vi "NI6363_CreateTasks.vi"(0 "tasks in":refnum<k21>[](array[refnum]), 1 "Camera Trigger":string="Dev1/ctr0", 2 "Exposure (s)":dbl=0.1 min=1.0 max=5000.0, 5 "Dye Settings":T1={"Dye Name"="", "Pulse Sequence"=[], "Emission Filter"=0, "Exposure (s)"=0.01, "Yellow Select"=FALSE, "# Pulses"=0} {"Exposure (s)" min=1.0 max=5000.0}, 7 "Sample Mode":T2(ring), 9 "Number of Samples":i32=100, 11 "error in":errorcluster) -> (4 "tasks out":refnum<k21>[](array[refnum]), 10 "Seq Length (s)":dbl, 15 "error out":errorcluster)   [LabVIEW 2010]
uses:
  <vilib>/DAQmx/write.llb/DAQmx Write (Digital 2D U32 NChan NSamp).vi
  <vilib>/DAQmx/write.llb/DAQmx Write (Analog 2D DBL NChan NSamp).vi
  <vilib>/daqmx/miscellaneous.llb/DAQmx Fill In Error Info.vi
  <vilib>/DAQmx/configure/trigger.llb/DAQmx Start Trigger (None).vi
  <vilib>/DAQmx/configure/timing.llb/DAQmx Timing (Implicit).vi
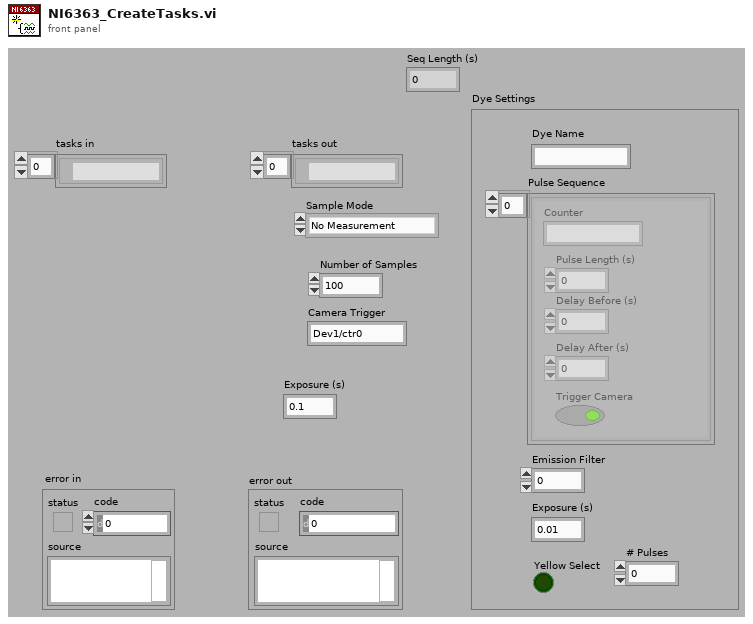
[diagram p1: front panel]
types:
  T1 = cluster{"Dye Name":string, "Pulse Sequence":cluster{"Counter":string, "Pulse Length (s)":dbl, "Delay Before (s)":dbl, "Delay After (s)":dbl, "Trigger Camera":bool}[], "Emission Filter":i16, "Exposure (s)":dbl, "Yellow Select":bool, "# Pulses":i32}
  T2 = enum16{"No Measurement", "Single Sample", "Continuous Samples", "N Samples"}
  T3 = cluster{"Counter":string, "Pulse Length (s)":dbl, "Delay Before (s)":dbl, "Delay After (s)":dbl, "Trigger Camera":bool}[]
  T4 = cluster{"Counter":string, "Pulse Length (s)":dbl, "Delay Before (s)":dbl, "Delay After (s)":dbl, "Trigger Camera":bool}
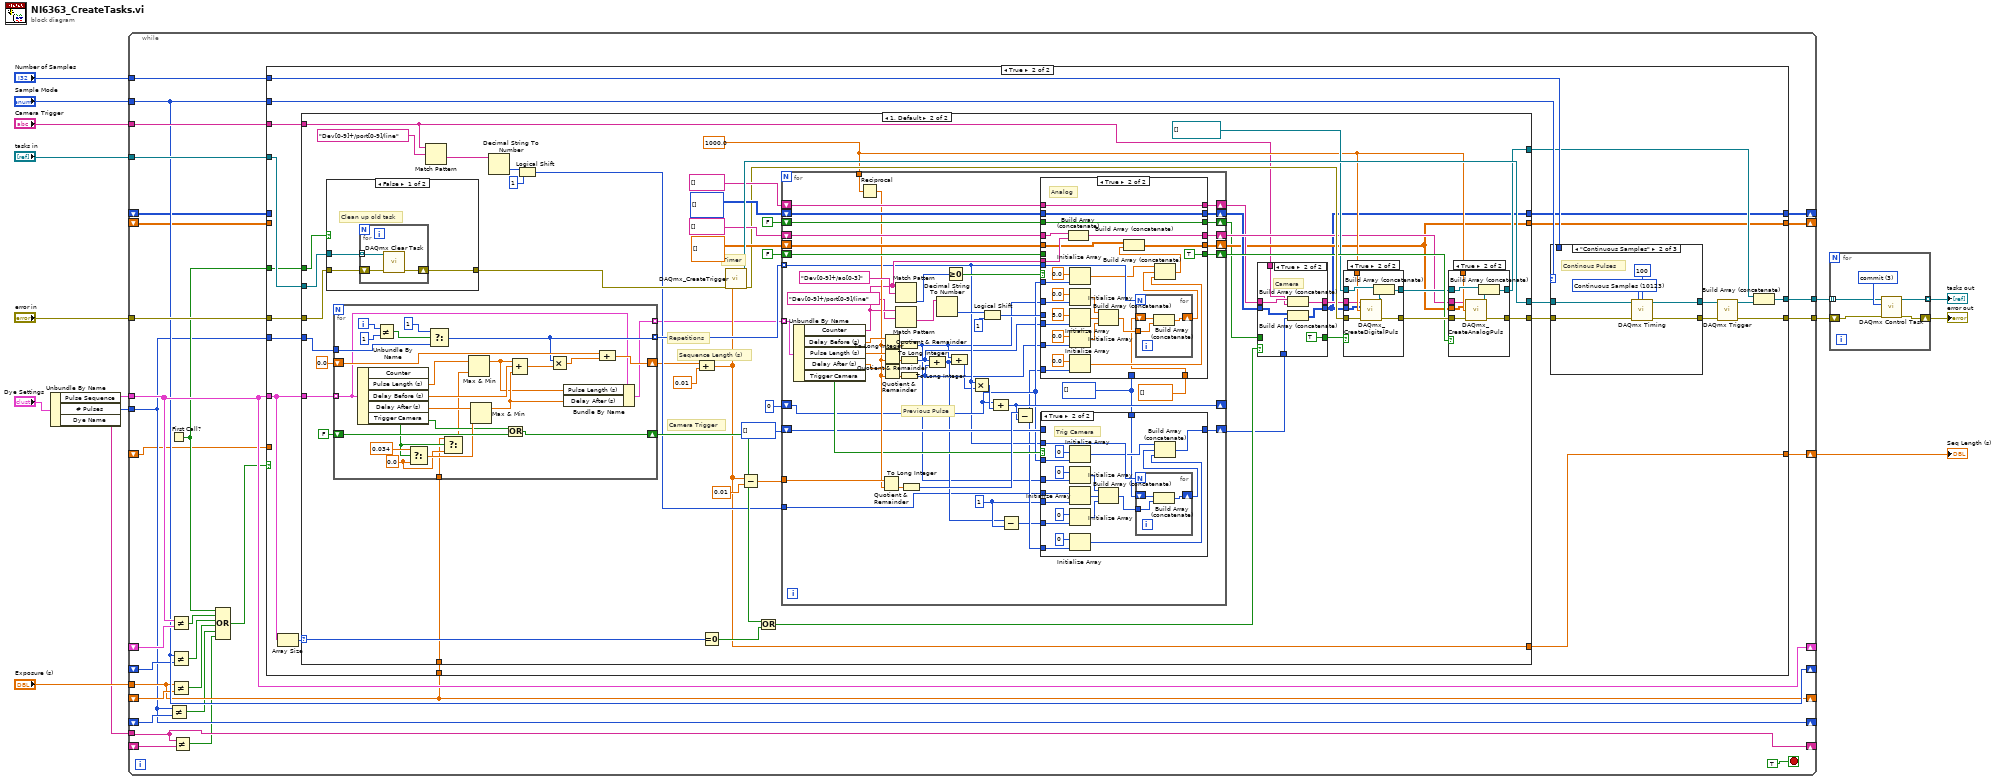
[diagram p0: block diagram]
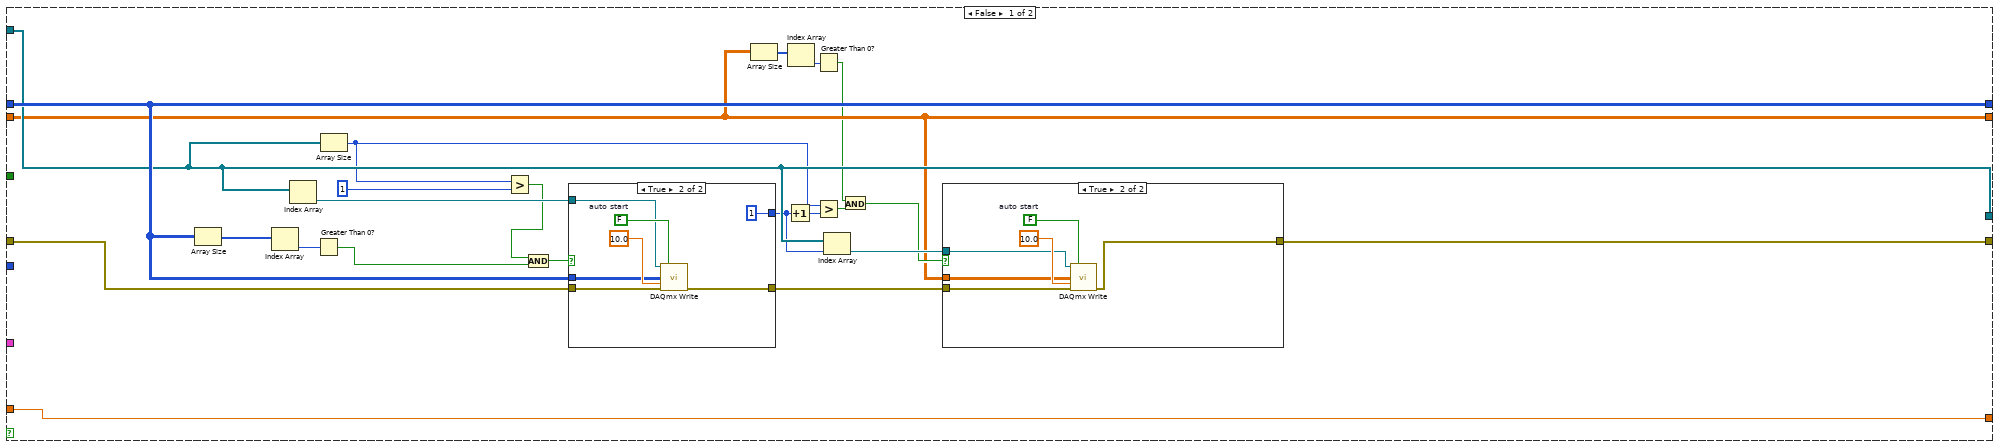
[diagram p2: hidden frame]
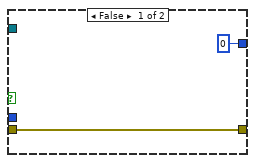
[diagram p4: hidden frame]
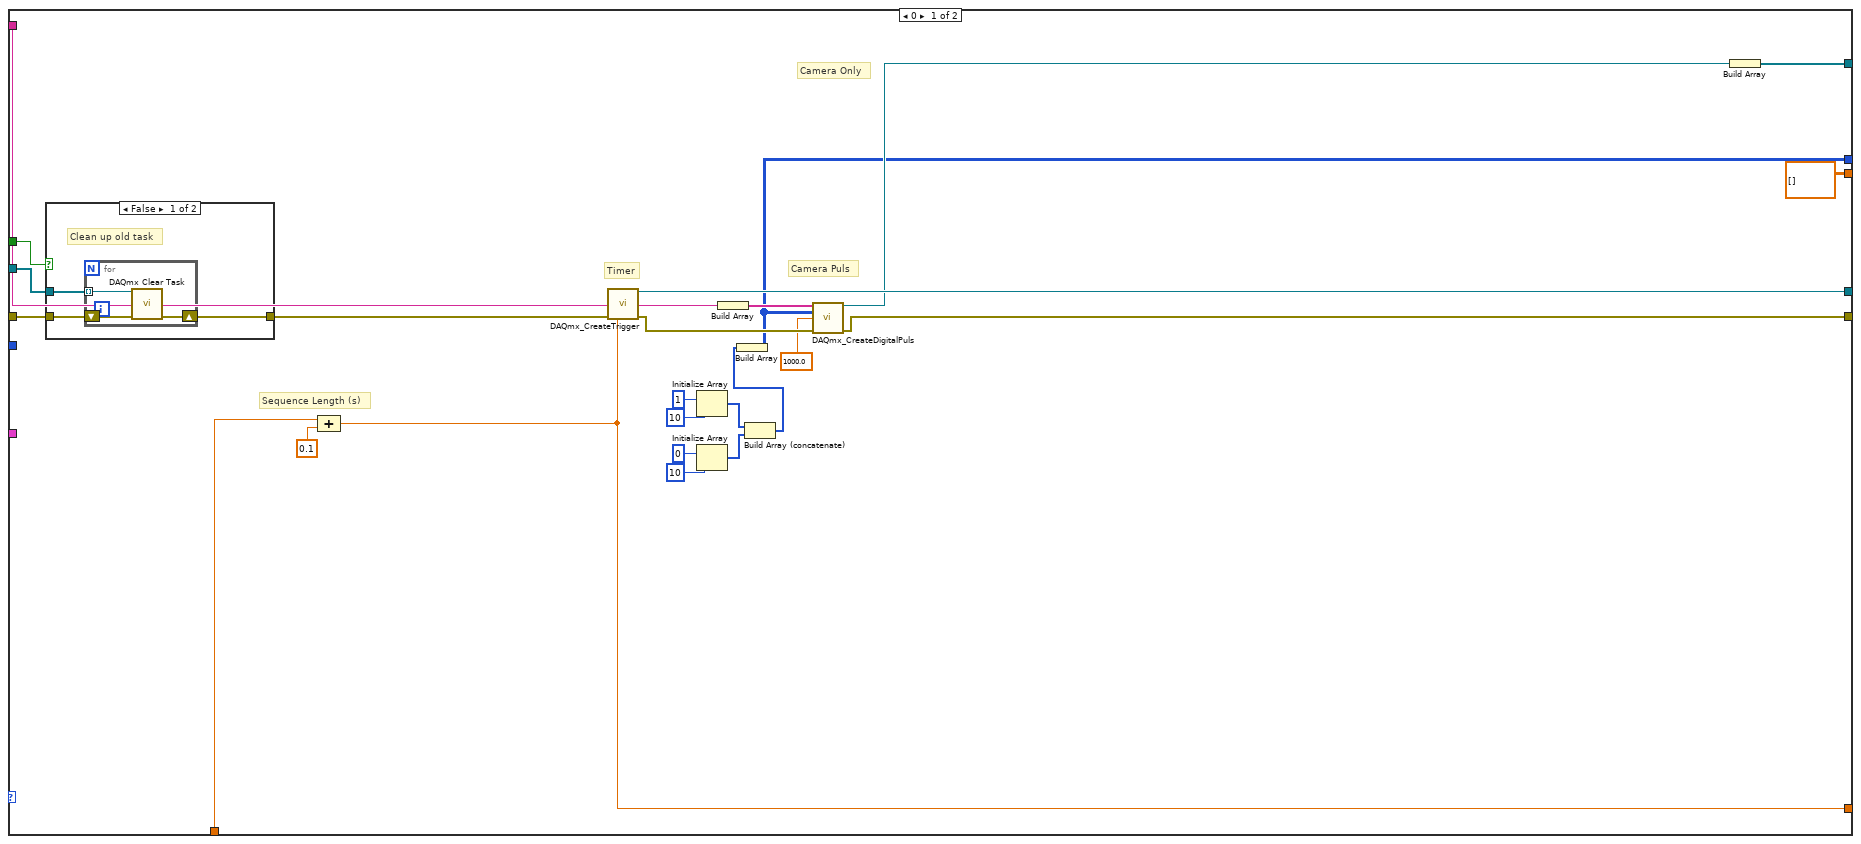
[diagram p5: hidden frame]
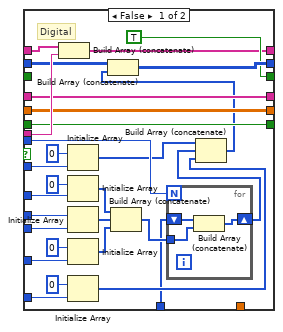
[diagram p12: hidden frame]
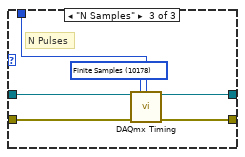
[diagram p14: hidden frame]
diagram:
  n1 = Unbundle By Name("Dye Settings") -> ("Pulse Sequence"=w9:T3, "# Pulses"=w8:i32, "Dye Name"=w2:string)
  n2 = while {
    tunnel: w9 -> [w38]
    tunnel: "Number of Samples" -> [w43]
    tunnel: "Camera Trigger" -> [w42]
    tunnel: "Sample Mode" -> [w33]
    tunnel: "error in" -> [w40]
    tunnel: [w44] -> w5
    tunnel: [w45] -> w6
    shift-right: [w38] -> _
    shift-left: _ -> [w39]
    tunnel: "tasks in" -> [w37]
    shift-right: [w33] -> _
    shift-left: _ -> [w32]
    tunnel: "Exposure (s)" -> [w29]
    shift-right: [w29] -> _
    shift-left: _ -> [w30]
    tunnel: w8 -> [w26]
    shift-right: [w26] -> _
    shift-left: _ -> [w28]
    shift-right: [w24] -> _
    shift-left: _ -> [w22]
    shift-right: [w23] -> _
    shift-left: _ -> [w21]
    tunnel: w2 -> [w19]
    shift-right: [w19] -> _
    shift-left: _ -> [w20]
    shift-right: [w17] -> w1
    shift-left: _ -> [w16]
    stop <- TRUE stop-if-true
    n3 = First Call?() -> (First Call?: T/F=w35:bool)
    n4 = Not Equal?(x=w26, y=w28) -> (x != y?=w27:bool)
    n5 = Not Equal?(x=w38, y=w39) -> (x != y?=w36:bool)
    n6 = Not Equal?(x=w33, y=w32) -> (x != y?=w34:bool)
    n7 = Not Equal?(x=w29, y=w30) -> (x != y?=w31:bool)
    n8 = Not Equal?(x=w19, y=w20) -> (x != y?=w18:bool)
    n9 = Compound Arithmetic op=OR(w35, w36, w34, w31, w27, w18) -> (w25:bool)
    n10 = case shown="True" w25 {
      tunnel: [w60 w91] -> w45
      tunnel: [w47 w103] -> w44
      tunnel: w43 -> [_ w102]
      tunnel: w42 -> [_ w100]
      tunnel: w33 -> [_ w99]
      tunnel: w40 -> [w68 w98]
      tunnel: w38 -> [_ w95]
      tunnel: w37 -> [w60 w97]
      tunnel: w35 -> [_ w96]
      tunnel: w29 -> [_ w94]
      tunnel: w26 -> [_ w92]
      tunnel: [w67 w87] -> w24
      tunnel: [w49 w86] -> w23
      tunnel: w22 -> [w67 _]
      tunnel: w21 -> [w49 _]
      tunnel: [w46 w85] -> w17
      tunnel: w16 -> [w46 _]
      frame False {
        n11 = Array Size(array=w67) -> (size(s)=w66:i32[])
        n12 = Index Array(array=w66) -> (element=w65:i32)  [unwired: 1 in]
        n13 = Index Array(array=w60) -> (element=w61:refnum<k21>)  [unwired: 1 in]
        n14 = Greater Than 0?(x=w65) -> (x > 0?=w64:bool)
        n15 = Array Size(array=w60) -> (size(s)=w55:i32)
        n16 = Greater?(x=w55, y=1) -> (0:w56:bool)
        n17 = And(x=w56, y=w64) -> (x .and. y?=w63:bool)
        n18 = case shown="True" w63 {
          tunnel: w68 -> [w77 w82]
          tunnel: w67 -> [_ w81]
          tunnel: [w77 w80] -> w62
          tunnel: [0 ("y") 1 ("y")] -> w53
          tunnel: w61 -> [_ w78]
          frame False {
          }
          frame True {
            w84 = FALSE  # auto start
            n19 = call-poly <vilib>:"DAQmx Write.vi"("task/channels in"=w78, "auto start"=w84, "data"=w81, "timeout"=10.0 ("timeout (s)"), "error in"=w82) -> ("error out"=w80:errorcluster)  [unwired: 8 in, 2 out]
          }
        }
        n20 = Array Size(array=w49) -> (size(s)=w51:i32[])
        n21 = Increment(x=w53) -> (x+1=w52:i32)
        n22 = Index Array(array=w51) -> (element=w50:i32)  [unwired: 1 in]
        n23 = Greater Than 0?(x=w50) -> (x > 0?=w48:bool)
        n24 = Greater?(x=w55, y=w52) -> (0:w58:bool)
        n25 = Index Array(array=w60, index=w53) -> (element=w59:refnum<k21>)
        n26 = And(x=w48, y=w58) -> (x .and. y?=w57:bool)
        n27 = case shown="True" w57 {
          tunnel: w62 -> [w69 w73]
          tunnel: w49 -> [_ w72]
          tunnel: w59 -> [_ w71]
          tunnel: [w69 w70] -> w47
          frame False {
          }
          frame True {
            w75 = FALSE  # auto start
            n28 = call-poly <vilib>:"DAQmx Write.vi"("task/channels in"=w71, "auto start"=w75, "data"=w72, "timeout"=10.0 ("timeout (s)"), "error in"=w73) -> ("error out"=w70:errorcluster)  [unwired: 8 in, 2 out]
          }
        }
      }
      frame True {
        n29 = Array Size(array=w95) -> (size(s)=w93:i32)
        n30 = case shown="1, Default" w93 {
          selector: w93 -> [_ w180]
          tunnel: [w110 w176] -> w101
          tunnel: w100 -> [w122 w145]
          tunnel: w98 -> [w129 w185]
          tunnel: w97 -> [w128 w184]
          tunnel: w96 -> [w127 w183]
          tunnel: w95 -> [_ w138]
          tunnel: w94 -> [w125 w139]
          tunnel: w92 -> [_ w152]
          tunnel: [w113 w178] -> w90
          tunnel: [w111 w165] -> w89
          tunnel: [w108 w155] -> w87
          tunnel: [dbl[][] [] w158] -> w86
          tunnel: [w106 w140] -> w85
          frame 0 {
            # "Timer"
            # "Camera Only"
            # "Camera Puls"
            # "Sequence Length (s)"
            n31 = case shown="False" w127 {
              tunnel: w129 -> [w131 w136]
              tunnel: [w132 w136] -> w124
              tunnel: w128 -> [w130 _]
              frame False {
                # "Clean up old task"
                n32 = for {
                  tunnel: w130 -> [w133] mode=indexing
                  shift-right: [w135] -> w132
                  shift-left: w131 -> [w134]
                  n33 = call <vilib>:"DAQmx Clear Task.vi"("task in"=w133, "error in"=w134) -> ("error out"=w135:errorcluster)  [unwired: 13 in]
                }
              }
              frame True {
              }
            }
            n34 = Compound Arithmetic op=ADD(w125, 0.1 ("Delay After (s) 2")) -> (w106:dbl)
            n35 = call "DAQmx_CreateTrigger.vi"("error in"=w124, "Sequence Length (s)"=w106) -> ("task out"=w113:refnum<k21>, "error out"=w123:errorcluster)  [unwired: 12 in]
            n36 = Initialize Array(u32 1 ("element"), 10 ("dimension size")) -> (w116:u32[])
            n37 = Initialize Array(u32 0 ("element"), 10 ("dimension size")) -> (w115:u32[])
            n38 = Build Array(w122) -> (w121:string[])
            n39 = Build Array (concatenate)(w116, w115) -> (w109:u32[])
            n40 = Build Array(w109) -> (w108:u32[][])
            n41 = call "DAQmx_CreateDigitalPuls.vi"("lines"=w121, "data"=w108, "rate"=1000.0, "error in"=w123) -> ("task out"=w112:refnum<k21>, "error out"=w110:errorcluster)  [unwired: 10 in]
            n42 = Build Array(w112) -> (w111:refnum<k21>[])
          }
          frame 1, Default {
            w164 = 1000.0 ("y")
            # "Repetitions"
            # "Timer"
            # "Camera Trigger"
            # "Sequence Length (s)"
            n43 = case shown="False" w183 {
              tunnel: w185 -> [w220 w225]
              tunnel: [w221 w225] -> w179
              tunnel: w184 -> [w219 _]
              frame False {
                # "Clean up old task"
                n44 = for {
                  tunnel: w219 -> [w222] mode=indexing
                  shift-right: [w224] -> w221
                  shift-left: w220 -> [w223]
                  n45 = call <vilib>:"DAQmx Clear Task.vi"("task in"=w222, "error in"=w223) -> ("error out"=w224:errorcluster)  [unwired: 13 in]
                }
              }
              frame True {
              }
            }
            n46 = for {
              tunnel: w138 -> [w368] mode=indexing
              shift-right: [w377] -> w142
              shift-left: 0.0 -> [w378]
              shift-right: [w389] -> w182
              shift-left: FALSE -> [w388]
              tunnel: w152 -> [w383]
              tunnel: [w374] -> w151 mode=indexing
              tunnel: w139 -> [w370]
              tunnel: [w367] -> w137 mode=indexing
              i -> [w385]
              w371 = 0.0 ("f")
              n47 = Unbundle By Name(w368) -> ("Pulse Length (s)"=w373:dbl, "Delay Before (s)"=w387:dbl, "Delay After (s)"=w380:dbl, "Trigger Camera"=w372:bool)  [unwired: 1 out]
              n48 = Not Equal?(x=w385, y=1 ("x")) -> (x != y?=w384:bool)
              n49 = Select(t=0.034 ("Delay After (s) 2"), s=w372, f=w371) -> (s? t:f=w379:dbl)
              n50 = Select(t=1, s=w384, f=w383) -> (s? t:f=w374:i32)
              n51 = Select(t=w370, s=w372, f=w371) -> (s? t:f=w369:dbl)
              n52 = Max & Min(x=w373, y=w369) -> (max(x,y)=w365:dbl)  [unwired: 1 out]
              n53 = Max & Min(x=w380, y=w379) -> (max(x,y)=w366:dbl)  [unwired: 1 out]
              n54 = Or(x=w372, y=w388) -> (x .or. y?=w389:bool)
              n55 = Compound Arithmetic op=ADD(w365, w387, w366) -> (w376:dbl)
              n56 = Multiply(x=w374, y=w376) -> (x*y=w375:dbl)
              n57 = Bundle By Name(cluster=w368, "Pulse Length (s)"=w365, "Delay After (s)"=w366) -> (w367:T4)
              n58 = Compound Arithmetic op=ADD(w378, w375) -> (w377:dbl)
            }
            n59 = Match Pattern(string=w145, regular expression="Dev[0-9]+/port[0-9]/line") -> (after substring=w147:string)  [unwired: 1 in, 3 out]
            n60 = Decimal String To Number(string=w147) -> (number=w146:i32)  [unwired: 2 in, 1 out]
            n61 = Logical Shift(y=w146, x=u32 1 ("element")) -> (x << y=w143:u32)
            n62 = Compound Arithmetic op=ADD(w142, 0.01 ("Delay After (s) 2")) -> (w140:dbl)
            n63 = Equal To 0?(x=w180) -> (x = 0?=w181:bool)
            n64 = call "DAQmx_CreateTrigger.vi"("error in"=w179, "Sequence Length (s)"=w140) -> ("task out"=w178:refnum<k21>, "error out"=w171:errorcluster)  [unwired: 12 in]
            n65 = Subtract(x=w140, y=0.01 ("Delay After (s) 2")) -> (x-y=w156:dbl)
            n66 = Or(x=w182, y=w181) -> (x .or. y?=w162:bool)
            n67 = for {
              tunnel: w137 -> [w276] mode=indexing
              shift-right: [w243] -> _
              shift-left: 0 -> [w239]
              tunnel: w156 -> [w267]
              shift-right: [w241] -> w149
              shift-left: u32[] [] -> [w240]
              shift-right: [w262] -> w163
              shift-left: string[] [] -> [w263]
              shift-right: [w264] -> w160
              shift-left: string[] [] -> [w265]
              shift-right: [w258] -> w159
              shift-left: u32[][] [] -> [w259]
              shift-right: [w260] -> w158
              shift-left: dbl[][] [] -> [w261]
              shift-right: [w257] -> w154
              shift-left: FALSE -> [w256]
              shift-right: [w255] -> w168
              shift-left: FALSE -> [w254]
              tunnel: w164 -> [w253]
              tunnel: w151 -> [w238] mode=indexing
              tunnel: w143 -> [w230]
              w228 = u32[] []
              w233 = 1
              # "Previous Pulse"
              n68 = Unbundle By Name(w276) -> ("Counter"=w251:string, "Delay Before (s)"=w275:dbl, "Pulse Length (s)"=w274:dbl, "Delay After (s)"=w227:dbl, "Trigger Camera"=w242:bool)
              n69 = Reciprocal(x=w253) -> (1/x=w252:dbl)
              n70 = Quotient & Remainder(x=w267, y=w252) -> (floor(x/y)=w266:dbl)  [unwired: 1 out]
              n71 = Quotient & Remainder(x=w275, y=w252) -> (floor(x/y)=w273:dbl)  [unwired: 1 out]
              n72 = Quotient & Remainder(x=w274, y=w252) -> (floor(x/y)=w272:dbl)  [unwired: 1 out]
              n73 = Quotient & Remainder(x=w227, y=w252) -> (floor(x/y)=w271:dbl)  [unwired: 1 out]
              n74 = Match Pattern(string=w251, regular expression="Dev[0-9]+/ao[0-3]") -> (offset past match=w270:i32)  [unwired: 1 in, 3 out]
              n75 = Match Pattern(string=w251, regular expression="Dev[0-9]+/port[0-9]/line") -> (after substring=w249:string)  [unwired: 1 in, 3 out]
              n76 = To Long Integer(number=w273) -> (32bit integer=w229:i32)
              n77 = To Long Integer(number=w272) -> (32bit integer=w236:i32)
              n78 = To Long Integer(number=w271) -> (32bit integer=w235:i32)
              n79 = To Long Integer(number=w266) -> (32bit integer=w244:i32)
              n80 = Compound Arithmetic op=ADD(w236, w235) -> (w231:i32)
              n81 = Decimal String To Number(string=w249) -> (number=w246:i32)  [unwired: 2 in, 1 out]
              n82 = Greater Or Equal To 0?(x=w270) -> (x >= 0?=w268:bool)
              n83 = Compound Arithmetic op=ADD(w229, w231) -> (w234:i32)
              n84 = Multiply(x=w238, y=w234) -> (x*y=w245:i32)
              n85 = Logical Shift(y=w246, x=u32 1 ("element")) -> (x << y=w247:u32)
              n86 = Compound Arithmetic op=ADD(w239, w245) -> (w243:i32)
              n87 = Subtract(x=w231, y=w233) -> (x-y=w232:i32)
              n88 = Subtract(x=w244, y=w243) -> (x-y=w237:i32)
              n89 = case shown="True" w268 {
                tunnel: w251 -> [w329 w361]
                tunnel: w265 -> [w317 w339]
                tunnel: [w316 w339] -> w264
                tunnel: w263 -> [w315 w341]
                tunnel: [w315 w340] -> w262
                tunnel: w261 -> [w328 w338]
                tunnel: [w328 w337] -> w260
                tunnel: w259 -> [w327 w336]
                tunnel: [w326 w336] -> w258
                tunnel: w236 -> [w320 w355]
                tunnel: [TRUE w335] -> w257
                tunnel: w256 -> [_ w335]
                tunnel: [w318 TRUE] -> w255
                tunnel: w254 -> [w318 _]
                tunnel: w247 -> [w314 _]
                tunnel: w239 -> [w312 w353]
                tunnel: w229 -> [w311 w352]
                tunnel: w235 -> [w310 w351]
                tunnel: w238 -> [w309 w350]
                tunnel: w237 -> [w303 w344]
                tunnel: w228 -> [w301 _]
                tunnel: dbl[] [] -> [_ w333]
                frame False {
                  # "Digital"
                  n90 = Build Array (concatenate)(w317, w329) -> (w316:string[])
                  n91 = Initialize Array(u32 0 ("element"), w312) -> (w307:u32[])
                  n92 = Initialize Array(u32 0 ("element"), w311) -> (w325:u32[])
                  n93 = Initialize Array(w314, w320) -> (w324:u32[])
                  n94 = Initialize Array(u32 0 ("element"), w310) -> (w323:u32[])
                  n95 = Initialize Array(u32 0 ("element"), w303) -> (w302:u32[])
                  n96 = Build Array (concatenate)(w325, w324, w323) -> (w308:u32[])
                  n97 = for {
                    N: w309 -> [_]
                    shift-right: [w331] -> w306
                    shift-left: w301 -> [w330]
                    tunnel: w308 -> [w332]
                    n98 = Build Array (concatenate)(w330, w332) -> (w331:u32[])
                  }
                  n99 = Build Array (concatenate)(w307, w306, w302) -> (w305:u32[])
                  n100 = Build Array (concatenate)(w327, w305) -> (w326:u32[][])
                }
                frame True {
                  # "Analog"
                  n101 = Build Array (concatenate)(w341, w361) -> (w340:string[])
                  n102 = Initialize Array(0.0 ("element"), w353) -> (w348:dbl[])
                  n103 = Initialize Array(0.0 ("element"), w352) -> (w360:dbl[])
                  n104 = Initialize Array(5.0 ("element"), w355) -> (w359:dbl[])
                  n105 = Initialize Array(0.0 ("element"), w351) -> (w358:dbl[])
                  n106 = Initialize Array(0.0 ("element"), w344) -> (w343:dbl[])
                  n107 = Build Array (concatenate)(w360, w359, w358) -> (w349:dbl[])
                  n108 = for {
                    N: w350 -> [_]
                    shift-right: [w363] -> w347
                    shift-left: w333 -> [w362]
                    tunnel: w349 -> [w364]
                    n109 = Build Array (concatenate)(w362, w364) -> (w363:dbl[])
                  }
                  n110 = Build Array (concatenate)(w348, w347, w343) -> (w346:dbl[])
                  n111 = Build Array (concatenate)(w338, w346) -> (w337:dbl[][])
                }
              }
              n112 = case shown="True" w242 {
                tunnel: w233 -> [_ w292]
                tunnel: w239 -> [_ w290]
                tunnel: w229 -> [_ w289]
                tunnel: w232 -> [_ w288]
                tunnel: w238 -> [_ w287]
                tunnel: w237 -> [_ w282]
                tunnel: [w277 w280] -> w241
                tunnel: w240 -> [w277 _]
                tunnel: w230 -> [_ w279]
                tunnel: w228 -> [_ w278]
                frame False {
                }
                frame True {
                  # "Trig Camera"
                  n113 = Initialize Array(u32 0 ("element"), w290) -> (w285:u32[])
                  n114 = Initialize Array(u32 0 ("element"), w289) -> (w297:u32[])
                  n115 = Initialize Array(w279, w292) -> (w296:u32[])
                  n116 = Initialize Array(u32 0 ("element"), w288) -> (w295:u32[])
                  n117 = Initialize Array(u32 0 ("element"), w282) -> (w281:u32[])
                  n118 = Build Array (concatenate)(w297, w296, w295) -> (w286:u32[])
                  n119 = for {
                    N: w287 -> [_]
                    shift-right: [w299] -> w284
                    shift-left: w278 -> [w298]
                    tunnel: w286 -> [w300]
                    n120 = Build Array (concatenate)(w298, w300) -> (w299:u32[])
                  }
                  n121 = Build Array (concatenate)(w285, w284, w281) -> (w280:u32[])
                }
              }
            }
            n122 = case shown="True" w162 {
              tunnel: [w191 w193] -> w155
              tunnel: w159 -> [w191 w195]
              tunnel: [w190 w197] -> w161
              tunnel: w160 -> [w190 w198]
              tunnel: w145 -> [_ w196]
              tunnel: w149 -> [_ w194]
              tunnel: w154 -> [w189 _]
              tunnel: [w189 TRUE] -> w153
              frame False {
              }
              frame True {
                # "Camera"
                n123 = Build Array (concatenate)(w198, w196) -> (w197:string[])
                n124 = Build Array (concatenate)(w195, w194) -> (w193:u32[][])
              }
            }
            n125 = case shown="True" w153 {
              tunnel: w171 -> [w210 w218]
              tunnel: [w210 w217] -> w177
              tunnel: refnum<k21>[] [] -> [w209 w216]
              tunnel: [w209 w214] -> w166
              tunnel: w164 -> [_ w213]
              tunnel: w161 -> [_ w212]
              tunnel: w155 -> [_ w211]
              frame False {
              }
              frame True {
                n126 = call "DAQmx_CreateDigitalPuls.vi"("lines"=w212, "data"=w211, "rate"=w213, "error in"=w218) -> ("task out"=w215:refnum<k21>, "error out"=w217:errorcluster)  [unwired: 10 in]
                n127 = Build Array (concatenate)(w216, w215) -> (w214:refnum<k21>[])
              }
            }
            n128 = case shown="True" w168 {
              tunnel: w177 -> [w200 w208]
              tunnel: [w200 w207] -> w176
              tunnel: w166 -> [w199 w206]
              tunnel: [w199 w204] -> w165
              tunnel: w164 -> [_ w203]
              tunnel: w163 -> [_ w202]
              tunnel: w158 -> [_ w201]
              frame False {
              }
              frame True {
                n129 = call "DAQmx_CreateAnalogPuls.vi"("physical channel"=w202, "data"=w201, "rate"=w203, "error in"=w208) -> ("task out"=w205:refnum<k21>, "error out"=w207:errorcluster)  [unwired: 10 in]
                n130 = Build Array (concatenate)(w206, w205) -> (w204:refnum<k21>[])
              }
            }
          }
        }
        n131 = case shown="\"Continuous Samples\"" w99 {
          tunnel: w101 -> [w390 w397 w403]
          tunnel: [w390 w396 w402] -> w105
          tunnel: w90 -> [w391 w395 w401]
          tunnel: [w391 w394 w400] -> w104
          tunnel: w102 -> [_ _ w398]
          frame "Single Sample", Default {
          }
          frame "Continuous Samples" {
            w393 = 10123 items=["Finite Samples"=10178, "Continuous Samples"=10123, "Hardware Timed Single Point"=12522] ("sample mode")
            # "Continous Pulses"
            n132 = call-poly <vilib>:"DAQmx Timing.vi"("task/channels in"=w395, "sample mode"=w393, "samples per channel"=100, "error in"=w397) -> ("task out"=w394:refnum<k21>, "error out"=w396:errorcluster)  [unwired: 10 in]
          }
          frame "N Samples" {
            w399 = 10178 items=["Finite Samples"=10178, "Continuous Samples"=10123, "Hardware Timed Single Point"=12522] ("sample mode")
            # "N Pulses"
            n133 = call-poly <vilib>:"DAQmx Timing.vi"("task/channels in"=w401, "sample mode"=w399, "samples per channel"=w398, "error in"=w403) -> ("task out"=w400:refnum<k21>, "error out"=w402:errorcluster)  [unwired: 10 in]
          }
        }
        n134 = call-poly <vilib>:"DAQmx Trigger.vi"("task/channels in"=w104, "error in"=w105) -> ("task out"=w88:refnum<k21>, "error out"=w103:errorcluster)  [unwired: 12 in]
        n135 = Build Array (concatenate)(w89, w88) -> (w91:refnum<k21>[])
      }
    }
  }
  "Seq Length (s)" <- w1
  n136 = for {
    tunnel: w6 -> [w407] mode=indexing
    shift-right: [w405] -> w4
    shift-left: w5 -> [w406]
    tunnel: [w404] -> w3 mode=indexing
    w408 = 3 items=["verify"=2, "reserve"=4, "commit"=3, "unreserve"=5, "abort"=6] ("action")
    n137 = call <vilib>:"DAQmx Control Task.vi"("task/channels in"=w407, "action"=w408, "error in"=w406) -> ("task out"=w404:refnum<k21>, "error out"=w405:errorcluster)  [unwired: 11 in]
  }
  "error out" <- w4
  "tasks out" <- w3
